vi "PNA3672B-H.vi"() -> ()   [LabVIEW 2018]
uses:
  <vilib>/Utility/file.llb/Write Delimited Spreadsheet (DBL).vi
panel:
  in  "Set Meter X":u16(ring) items=["PMMS field  0", "PPMS temp  1", "PPMS angle 2"]
  in  "Rate":dbl=50.0
  in  "Scan type":u16(ring)=1 items=["sweep  0", "liner  1"]
  in  "Int Rate (Oe/s)\nRate()":dbl=200.0 format="%#_13g"
  in  "Int Delay":dbl=5.0
  in  "Measurement Type":i32(ring)=2 items=["S11", "S12", "S21", "S22", "A", "B", "R1", "R2", "A/B", "B/A"]
  in  "Sweep Points (801)":i32=401
  in  "Stop Freq (26.4 E+9)":dbl=10000000000.0 format="%.2p"
  in  "Start Freq (10.0 E+6)":dbl=5000000000.0 format="%.2p"
  in  "?":enum32{"S-parameter", "Phase"}(tab)
  out "?":dbl[](graph)=[-5.13992176013, -5.77985062144, -7.16807133092, -9.42108029997, -10.1399493654, -8.71596720045, -7.83267897782, -7.42919537856, -6.76032356605, -6.18585704171, -5.97046539483, -5.73016109242, -5.37263627886, -5.1017928619, -5.00368082967, -5.17829909409, -5.80323496787, -7.15574927433, -8.9987014472, -9.38466845211, -8.49380537991, -7.97106763789, -7.32574501548, -6.50085765669, -6.07911357188, -5.85829530019, -5.55446508735, -5.36941855458, -5.36021729011, -5.31851913016, -5.5643037132, -6.25259294468, -7.43240745282, -9.04614952431, -9.99905930623, -9.4413228677, -8.04418422737, -6.84363600252, -6.40371174912, -6.24462050869, -5.56869109258, -4.87352825858, -4.66321212934, -4.69307312429, -4.7591466358, -5.14591077224, -5.89876799636, -7.07657010714, -8.54625263275, -9.49167159085, -9.24509469713, -8.19081925887, -7.18917811597, -6.67042363043, -6.07630869368, -5.34692013326, -4.941337791, -4.84078157888, -4.73147936533, -4.79218794585, -5.14409746704, -5.78112817858, -6.86212442292, -8.05457821576, -8.81261762726, -8.79759046484, -7.92763479317, -6.85071777851, -6.21538876741, -5.77195549778, -5.33268495617, -5.03854648325, -4.88320527288, -4.92756756489, -5.11628322032, -5.50972588621, -6.30511280642, -7.56416681135, -8.3419108514, -8.66657669285, -8.81033918175, -8.33720970709, -7.27317631141, -6.37575047564, -5.75176099873, -5.26236758865, -4.89247637429, -4.65199723878, -4.64290261895, -4.80678031934, -5.27987797209, -6.19570891325, -7.17215718437, -7.74510640519, -8.53976798715, -8.98978028998, -8.64998426925, -7.70133626893, -6.94492286579, -6.39681487173, -5.94202187224, -5.51750467546, -5.20454435892, -5.09708374418, -5.13935702712, -5.44519548006, -6.11037282184, -6.71822270524, -7.21836141914, -7.75556602746, -7.94679767326, -7.58810236429, -7.11458256386, -6.64461014107, -6.17815328806, -5.82869822125, -5.58855306212, -5.47932972608, -5.57017360045, -5.73509999009, -6.10279430727, -6.65628309091, -7.20691574144, -7.75099153049, -8.14236217319, -7.98342278217, -7.63567730066, -7.37171742701, -6.93968192443, -6.37024086203, -5.917649598, -5.55597456297, -5.30308721864, -5.25401060366, -5.39488001063, -5.74026002176, -6.23480440616, -6.7661133476, -7.41657074229, -7.91867432885, -8.02300874345, -8.08809276389, -7.99786036781, -7.59075128208, -7.08210024901, -6.64548196863, -6.30005305904, -6.11058253071, -6.07953628099, -6.16464230657, -6.4216011742, -6.75039933455, -7.09214315299, -7.52704057997, -7.86129689791, -7.85671742728, -7.68286255005, -7.41290778429, -7.08377575548, -6.76583315521, -6.51875926079, -6.34242015251, -6.29759006079, -6.28815023049, -6.49115089113, -6.90636491421, -7.42097777053, -7.82869609191, -8.25316429775, -8.57203674825, -8.66045753728, -8.58510840229, -8.34411171176, -8.02714571689, -7.70639713953, -7.43771426738, -7.29138512983, -7.25008195523, -7.33202806195, -7.54992861785, -7.91918366742, -8.29162811805, -8.70581027915, -9.12417570214, -9.40804943396, -9.52932859893, -9.52034892046, -9.35525338025, -9.1032378942, -8.86236246566, -8.66294128383, -8.56510147029, -8.56774273254, -8.68410230266, -8.89739073051, -9.14323997619, -9.40506155611, -9.67348671236, -9.91088070103, -10.0542110985, -10.1095993532, -10.0803215484, -9.93148871528, -9.72256956142, -9.5147582593, -9.31823788768, -9.17445611494, -9.08113535802, -9.05167488482, -9.03923798355, -9.03083138808, -8.97910059153, -8.88873008249, -8.75205020612, -8.56332184176, -8.38303089171, -8.22071675953, -8.1326945275, -8.05324942924, -8.05991169849, -8.05283861322, -8.16061412627, -8.29991125623, -8.47313413203, -8.57827792821, -8.65705773799, -8.67162556802, -8.6057904591, -8.47009108033, -8.25729780045, -8.0152070315, -7.7655926039, -7.57485266834, -7.4910467002, -7.5129644452, -7.59557810152, -7.73661469714, -7.87778576133, -7.99771913554, -8.13288701393, -8.32119654517, -8.46279170426, -8.35203711312, -8.15020651839, -7.88837024277, -7.57982328212, -7.34318110093, -7.19136752754, -7.15618430333, -7.21185640414, -7.36077780873, -7.56529300929, -7.83073868392, -8.06774468869, -8.2351880619, -8.33762695258, -8.31073052943, -8.14118362882, -7.90375456362, -7.61723861488, -7.2588078898, -6.98083255383, -6.72776846318, -6.63447620124, -6.71988359154, -6.77368052089, -7.11144857387, -7.37229013114, -7.68932033478, -7.98689247769, -8.19760417787, -8.28714274409, -8.23062581971, -8.04937534418, -7.79579768498, -7.49888178556, -7.14573710276, -6.8922594941, -6.68162816217, -6.62820636947, -6.6955037322, -6.78307910466, -7.05744034392, -7.40195880161, -7.7574756049, -8.08037713376, -8.15070297057, -8.18821061526, -8.11423800124, -8.14165480442, -7.82050654127, -7.70209407804, -7.46090411593, -7.38273407697, -7.28868801655, -7.2807538442, -7.37534790317, -7.51701471023, -7.62436761408, -7.74089685338, -7.80383275981, -7.78343031545, -7.69515063327, -7.53178482724, -7.31402064896, -7.10952415038, -6.93928420782, -6.83727474814, -6.81097857553, -6.86779731028, -6.98749866679, -7.1971793431, -7.38247926971, -7.54210372946, -7.63862857053, -7.6778904201, -7.62271286134, -7.51451127096, -7.34315098363, -7.14136947685, -6.96438816881, -6.79121451838, -6.69070621876, -6.65869471212, -6.6568027501, -6.72643653407, -6.75786124102, -6.84265238932, -6.87777149766, -6.88558318069, -6.83848750817, -6.77553827667, -6.73350349871, -6.65482701872, -6.61622596932, -6.6129050715, -6.66890540435, -6.75901895758, -6.87042004371, -6.99510404698, -7.12635533618, -7.23896129909, -7.3018797066, -7.30472334689, -7.2278149539, -7.12604877595, -6.99605011464, -6.87128470585, -6.7482182436, -6.68177936196, -6.64596095095, -6.67518331249, -6.72354301906, -6.76504258436, -6.82319955092, -6.88612600955, -6.96369683881, -6.96338059421, -6.94981925867, -6.96403414884, -7.03463520635, -7.05139105632, -7.06288523133, -7.13843539676, -7.23109085353, -7.37977824355, -7.53461754848, -7.69673249323, -7.72378467103, -7.5683548814, -7.38247183674, -7.21553067591, -7.04830148594, -6.7342671306, -6.48401257302, -6.32864044001, -6.26546650427, -6.27421138562, -6.39994502813, -6.65464294869, -7.02210039821, -7.43592259732, -7.79248421008, -7.98611288379, -7.936089008, -7.72371617285, -7.43734298033, -7.08800620268, -6.70804913045, -6.40077439135, -6.20272644312, -6.08472382437, -6.05534323724, -6.16756242594, -6.45803936543, -6.94832314698, -7.53318826156, -8.1920689104, -8.83012599835, -8.93751078087, -8.51422059906]
  in  "Format 1":string(combo)="IMAGinary"
  out "Sweep Time":dbl=0.19447074 format="%.2p"
  out "强度图":dbl[][](graph)
  out "?":dbl[](graph)=[32.7315489441, -56.8824930209, -156.803721114, 88.5947580109, -30.9871374098, -141.449771615, 121.640209048, 37.6741293404, -40.8852651853, -119.359692213, 163.750895669, 88.8384574151, 13.3240499463, -63.9260096883, -143.405981865, 133.50983641, 44.7073194162, -53.5440511171, -162.601840619, 79.6102257103, -33.2172204397, -129.587126545, 146.770832642, 66.0878076236, -13.5370500567, -90.5924606956, -167.123471558, 115.554059762, 38.2283746273, -41.0001051979, -124.5184635, 147.282505129, 51.2497788989, -55.3731568606, -169.072027126, 83.656838734, -12.3021295083, -102.452717622, 172.324212586, 94.0523173761, 18.2165179889, -60.6156999542, -140.290937488, 140.810952688, 60.5738116612, -22.7172481731, -109.652017526, 157.110661295, 55.5866667056, -53.048087914, -159.690576715, 102.426242104, 10.9688911141, -74.6158856148, -155.081353888, 124.521714604, 43.6872727344, -35.7101270301, -114.590575382, 164.575544825, 82.0901426192, -3.95730226738, -95.0285928659, 167.794680235, 63.4588246527, -41.3214166135, -139.542029674, 127.111889367, 38.4815112044, -45.3547081312, -126.698352397, 152.651043355, 72.8446050682, -7.32560497409, -87.954289903, -171.230817426, 102.154808567, 13.2571754957, -79.6451209514, 178.303953923, 74.3792037792, -23.0304688081, -115.678534016, 154.832081054, 69.078005824, -13.7902174538, -95.1617582494, -176.131266186, 102.595765505, 20.070955094, -64.77731603, -151.901641013, 120.060177573, 25.9178457946, -74.1552255377, -172.122975555, 94.1815920909, 2.03725084929, -87.9142000741, -174.423581853, 101.589486571, 18.9341666675, -63.971438346, -147.051928699, 128.678423861, 42.0808306788, -46.0050808644, -135.731355716, 130.13457169, 33.6068897418, -61.4897176925, -155.108417403, 113.175505949, 24.5315133942, -62.1326199724, -147.488272424, 128.115000927, 43.7882921958, -40.6090269269, -125.642775982, 147.354518001, 58.9206602667, -31.5941239859, -124.861969493, 141.766872237, 48.291882116, -45.4663429063, -136.890884056, 135.083717726, 47.7746115954, -38.6603639921, -124.258719066, 150.511571612, 65.2257451029, -20.5321047268, -107.529724429, 163.858540461, 72.6260181241, -20.7889524121, -113.818227096, 152.538492755, 58.8294740517, -31.932569054, -119.679705811, 153.414625818, 67.9360203075, -16.761149864, -101.241236752, 174.044379129, 88.3204159639, 0.878356230139, -88.3268956559, 179.63752201, 85.3637790641, -9.034868342, -103.096223064, 163.658409742, 72.8031961431, -15.6688017348, -102.22000084, 172.884816589, 88.5456131454, 4.55185396442, -80.2707904752, -166.719177803, 105.182195151, 16.096076312, -75.3026072059, -168.714844573, 97.6383537905, 4.33654879439, -87.7067545736, -177.84505287, 93.8380017628, 6.97761796918, -78.9002782548, -164.400040415, 110.116141956, 24.0091146464, -62.9948301844, -150.732269265, 120.632831154, 30.5535960961, -60.2411898127, -151.292645694, 117.497721205, 26.9689156873, -62.5301818212, -151.367772947, 120.685035314, 33.3394512614, -53.5091290058, -140.068434299, 133.595476642, 47.2881570478, -39.0864346002, -125.960768837, 146.612134326, 58.7129453948, -29.8143369144, -118.986171156, 151.549019718, 61.9477483812, -27.6598757887, -116.976616287, 154.302945475, 66.1878564391, -21.2904270435, -108.127149698, 165.52171244, 79.4590872768, -6.83103821612, -93.6121690666, 178.732349126, 90.3652078735, 1.14449863919, -88.5963134199, -178.65967342, 91.3537131772, 1.69568242194, -87.743176037, -176.928296806, 94.3550205229, 6.14869585327, -81.7831524664, -169.539688075, 102.802172688, 15.0397411523, -72.8651220086, -160.916924229, 110.823595481, 22.527364207, -65.9275903187, -154.288949487, 117.446350182, 28.9943452624, -59.7324147838, -148.897831038, 121.577481918, 31.6490376728, -58.2592650543, -147.677831112, 123.372313971, 35.0181759661, -52.4179118064, -139.26608448, 134.01427806, 47.4191105099, -39.5141347671, -126.836073187, 144.949439688, 55.7351697066, -34.3928698653, -125.099446067, 143.632754958, 52.5752734821, -37.7294449644, -127.148944827, 144.53035721, 57.5778533047, -28.887570595, -114.999609647, 158.525366628, 71.0429767896, -15.3772796346, -103.919515773, 166.689371892, 77.0093180077, -13.7911821267, -104.825362398, 164.200014669, 74.3696417703, -14.7668942558, -102.967824914, 169.411234659, 82.6122419887, -4.39400690011, -91.4543478077, -178.76858485, 93.3771862952, 4.85591617141, -84.3294425775, -173.865576593, 96.3465827134, 6.2490852757, -83.2265580877, -173.015984117, 97.78007546, 8.28655359163, -79.76381321, -167.927920395, 105.464735796, 17.261076543, -70.0043839303, -157.791686994, 114.069074987, 25.2581831541, -63.7608616106, -153.623185239, 116.145683725, 25.8986335399, -64.2331220915, -154.057904631, 116.747887891, 28.1083515487, -59.9530342147, -147.477795048, 125.430845568, 38.358901893, -48.7756883964, -136.513013638, 135.090000778, 45.9410900506, -44.132522883, -134.81386025, 134.272943326, 43.463402508, -47.1014527938, -136.910600874, 134.009988341, 45.6836835135, -41.9002560197, -129.524645098, 143.209830004, 55.3766093333, -32.4089929655, -121.157084902, 149.743492126, 60.2247754669, -29.3814603663, -118.881768282, 151.742455687, 62.7529965091, -25.7990392292, -114.353341921, 157.350941943, 68.9119611723, -19.6248853555, -108.53843891, 162.242639238, 72.8768930287, -16.4662361825, -105.666386314, 165.419060839, 76.7648920544, -11.5379476172, -99.5758100655, 172.435108019, 84.1025390815, -4.88019096974, -94.3024874425, 175.738534312, 85.5960595678, -4.7695105397, -94.9315233658, 175.485146261, 86.9188499232, -0.563780453117, -87.6986696312, -174.426390626, 99.1825213591, 13.1552601395, -74.0907708672, -162.246232711, 108.15987703, 17.2417782382, -74.8265647472, -167.397054628, 100.744515615, 9.42910460872, -80.8444801244, -169.303652166, 104.659034338, 19.8043132765, -65.0554301395, -149.709685307, 125.555931464, 40.1202806793, -46.5671247267, -134.968163745, 134.5694261, 41.8189582943, -52.9338270423, -148.539509551, 116.764065214, 24.1899149115, -65.4304007989, -152.041950572, 122.95863872, 39.038287934, -44.0062424284, -126.556835392, 150.597800658, 66.9189093569, -18.4084130856, -105.815690398, 163.407074758, 67.8515876273, -29.9904541232, -128.522871427, 135.807686]
  in  "Format 2":string(combo)="PHASe"
  out "强度图 2":dbl[][](graph)
  out "VISA 2":refnum<visa-resource-name>="GPIB0::16::INSTR"
  out "Time(s)":dbl=21.755
  out "Current H (Oe)":dbl=19.0 format="%.4g"
  in  "File":string="Hello"
  in  "Directory":string="D:\\ff"
  out "file":path=path "E:/ff/Hello@_100ms_1.txt"
  in  "wait":u32=400
  out "Hset":dbl[](array[numeric])=[14.0, 14.5, 15.0, 15.5, 16.0, 16.5, 17.0, 17.5, 18.0, 18.5, 19.0]
  in  "L/S":enum32{"Loop", "Scan"}(radio)=enum."Scan"
  in  "停止":bool
  in  "Hpara":dbl[][](array[numeric])=[[-1000.0, 1000.0, 10.0], [0.0, 0.0, 0.0], [0.0, 0.0, 0.0], [0.0, 0.0, 0.0], [0.0, 0.0, 0.0], [0.0, 0.0, 0.0], [0.0, 0.0, 0.0], [0.0, 0.0, 0.0], [0.0, 0.0, 0.0], [0.0, 0.0, 0.0], [0.0, 0.0, 0.0], [0.0, 0.0, 0.0], [0.0, 0.0, 0.0]] caption="Hi(Oe)     Hf(Oe)   Steps"
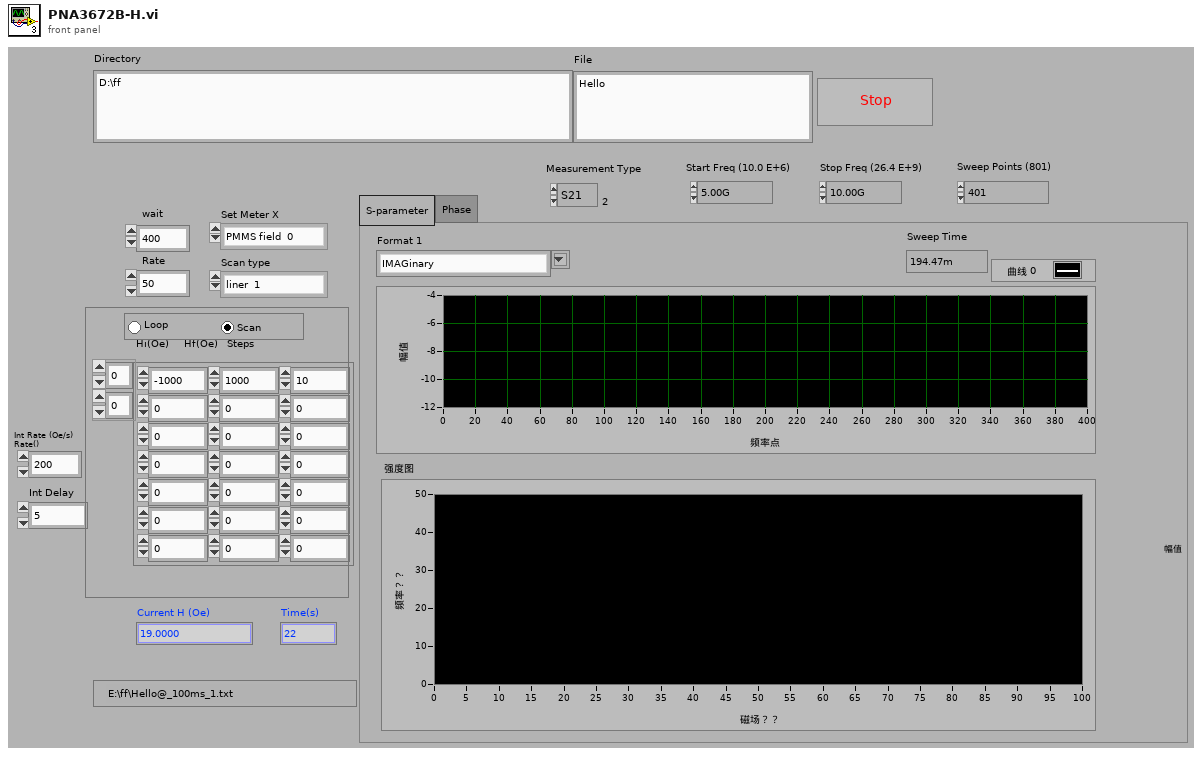
[diagram p1: front panel]
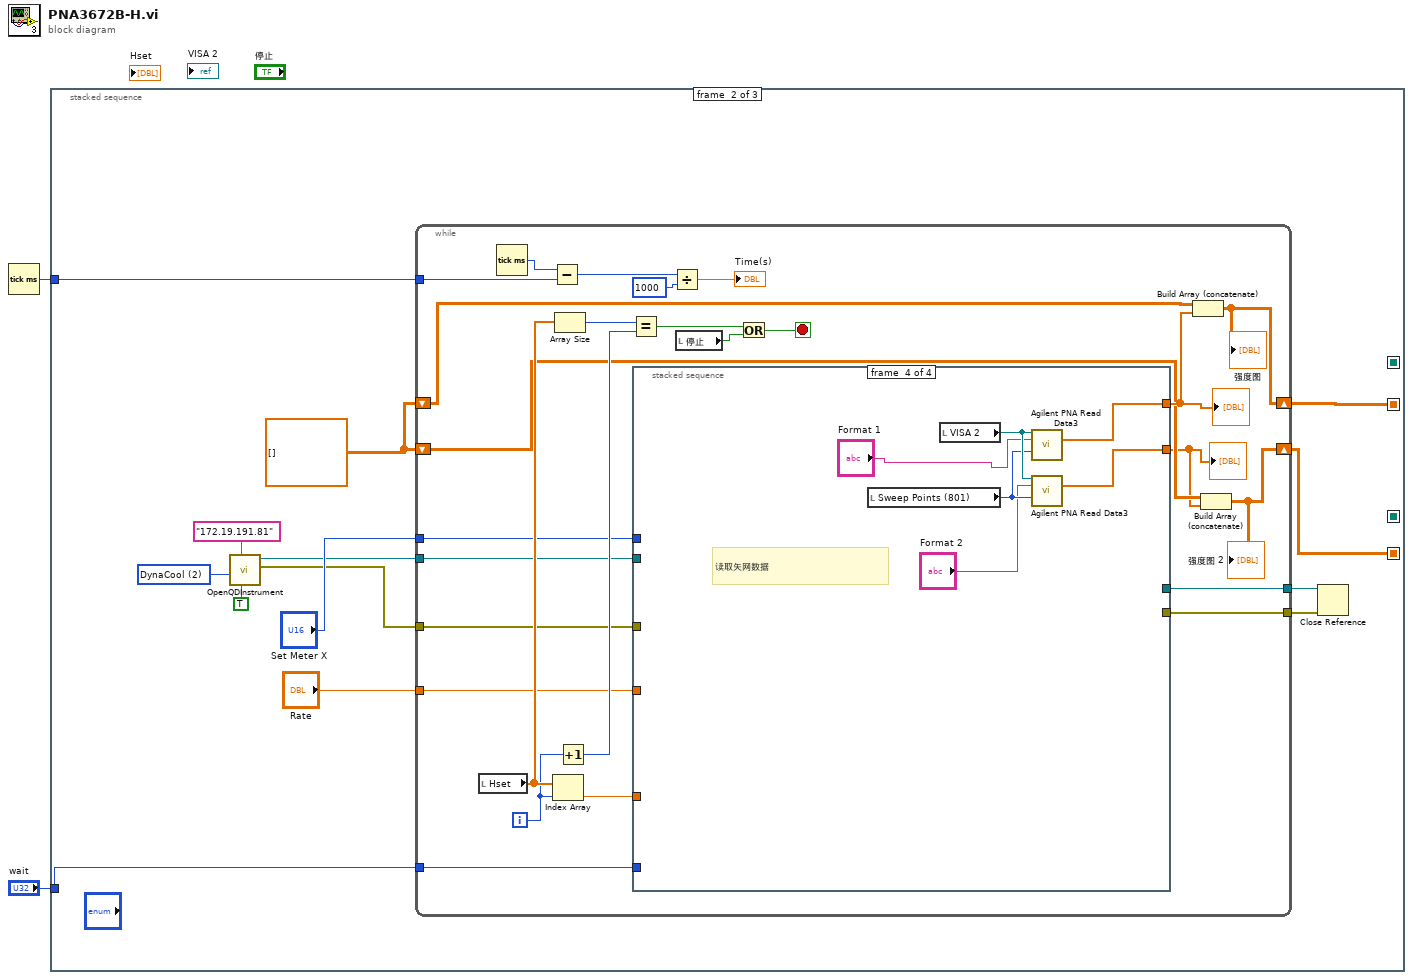
[diagram p0: block diagram]
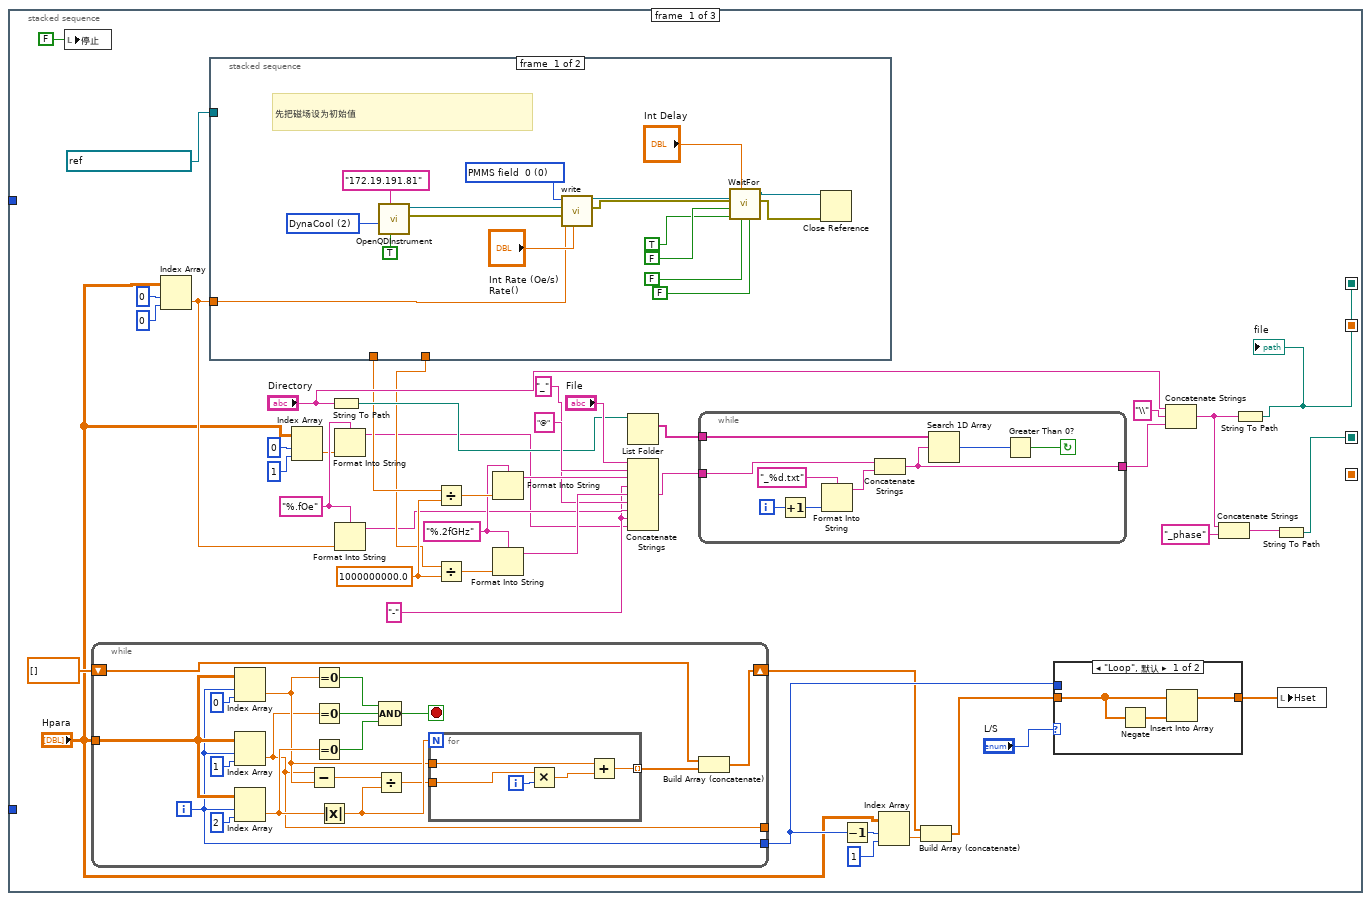
[diagram p2: hidden frame]
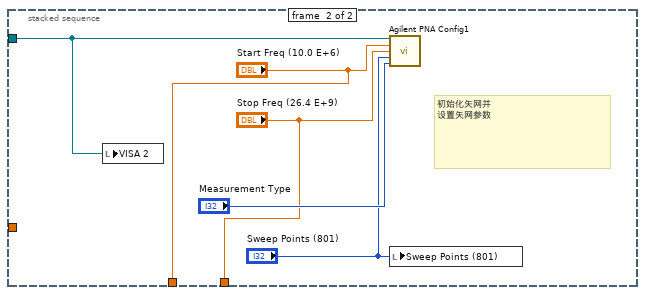
[diagram p3: hidden frame]
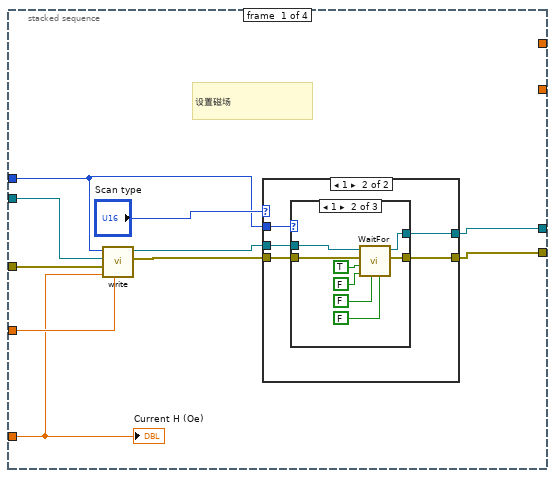
[diagram p5: hidden frame]
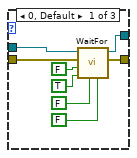
[diagram p7: hidden frame]
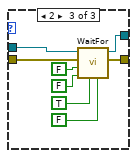
[diagram p8: hidden frame]
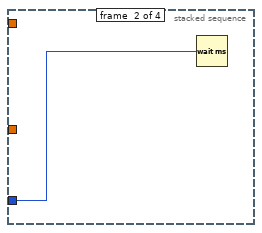
[diagram p9: hidden frame]
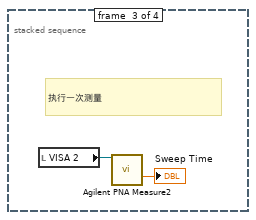
[diagram p10: hidden frame]
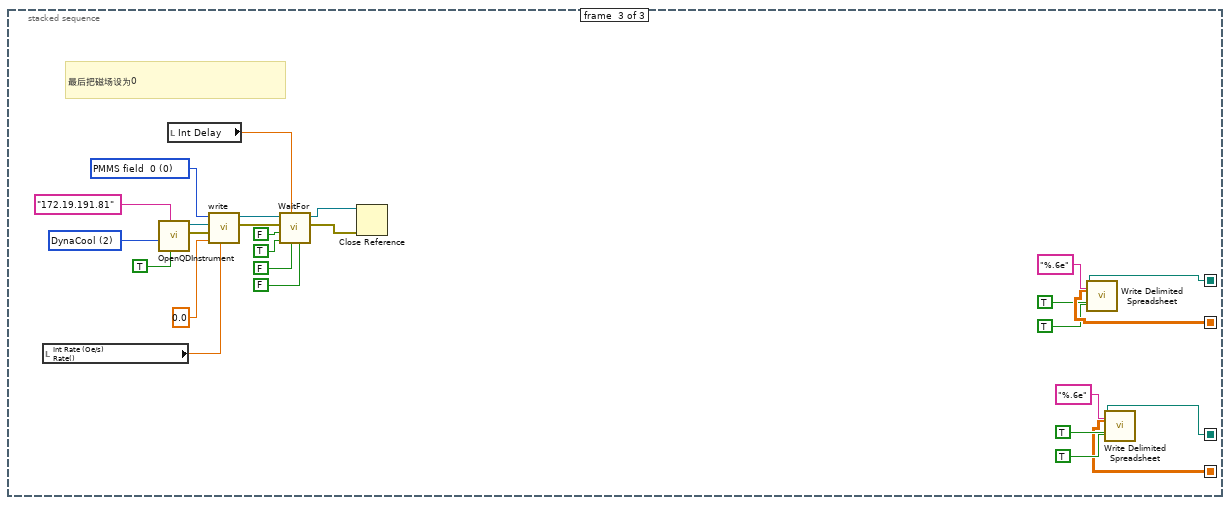
[diagram p11: hidden frame]
diagram:
  n1 = Tick Count (ms)() -> (millisecond timer value=w2:u32)
  n2 = stacked-sequence {
    seq-local: [_ w115 _] -> [_ _ w219]
    seq-local: [w35 _ _] -> [_ _ w221]
    seq-local: [w3 _ _] -> [_ _ w196]
    seq-local: [_ w105 _] -> [_ _ w195]
    tunnel: w2 -> [_ w118 _]
    tunnel: "wait" -> [_ w117 _]
    frame #0 {
      w9 = "%.fOe" ("格式字符串")
      w13 = "-" ("字符串")
      w20 = 1000000000.0 ("y")
      w21 = "%.2fGHz" ("格式字符串")
      n3 = local write "停止"(FALSE ("停止")) -> ()
      n4 = while {
        tunnel: "Hpara" -> [w92]
        shift-right: [w85] -> w29
        shift-left: dbl[] [] -> [w84]
        tunnel: [w83] -> _
        tunnel: [w82] -> w31
        i -> [w82]
        stop <- w96 stop-if-true
        n5 = Index Array(array=w92, index (row)=w82, index (col)=0 ("禁用的索引 (col)")) -> (element=w87:dbl)
        n6 = Index Array(array=w92, index (row)=w82, index (col)=1 ("禁用的索引 (col)")) -> (element=w83:dbl)
        n7 = Index Array(array=w92, index (row)=w82, index (col)=2 ("禁用的索引 (col)")) -> (element=w91:dbl)
        n8 = Subtract(x=w83, y=w87) -> (x-y=w90:dbl)
        n9 = Equal To 0?(x=w87) -> (x = 0?=w99:bool)
        n10 = Equal To 0?(x=w83) -> (x = 0?=w98:bool)
        n11 = Equal To 0?(x=w91) -> (x = 0?=w97:bool)
        n12 = Absolute Value(x=w91) -> (abs(x)=w89:dbl)
        n13 = Divide(x=w90, y=w89) -> (x/y=w88:dbl)
        n14 = Compound Arithmetic op=AND(w99, w98, w97) -> (w96:bool)
        n15 = for {
          N: w89 -> [_]
          tunnel: [w104] -> w86 mode=indexing
          tunnel: w88 -> [w101]
          tunnel: w87 -> [w100]
          i -> [w103]
          n16 = Multiply(x=w101, y=w103) -> (x*y=w102:dbl)
          n17 = Add(x=w100, y=w102) -> (x+y=w104:dbl)
        }
        n18 = Build Array (concatenate)(w84, w86) -> (w85:dbl[])
      }
      n19 = Index Array(array="Hpara", index (row)=0 ("索引 (行)"), index (col)=0 ("禁用的索引 (col)")) -> (element=w15:dbl)
      n20 = stacked-sequence {
        tunnel: refnum<visa-resource-name> "GPIB0::16::INSTR" ("VISA资源名称") -> [_ w66]
        tunnel: w15 -> [w49 _]
        tunnel: [_ "Start Freq (10.0 E+6)"] -> w24
        tunnel: [_ "Stop Freq (26.4 E+9)"] -> w19
        frame #0 {
          w58 = u16 0 items=["PMMS field  0", "PPMS temp  1", "PPMS angle 2"] ("Set Meter")
          w61 = 2 items=["PPMS", "VersaLab", "DynaCool", "SVSM"] ("Instrument\nType")
          # "先把磁场设为初始值"
          n21 = call "OpenQDInstrument.vi"("Remote"=TRUE, "IP Address"="172.19.191.81", "Instrument Type"=w61) -> ("error out"=w59:errorcluster, "Instrument Ref"=w60:refnum<k24>)  [unwired: 5 in]
          n22 = call "write.vi"("Rate"="Int Rate (Oe/s)\nRate()", "value"=w49, "error in (no error)"=w59, "Instrument Ref In"=w60, "Set Meter"=w58) -> ("error out"=w56:errorcluster, "Instrument Ref Out"=w55:refnum<k24>)  [unwired: 5 in]
          n23 = call "WaitFor.vi"("Wait For Chamber"=FALSE, "Wait For Position"=FALSE, "Delay"="Int Delay", "Wait For Field"=TRUE, "Wait For Temperature"=FALSE, "error in (no error)"=w56, "Instrument Ref In"=w55) -> ("error out"=w47:errorcluster, "Instrument Ref Out"=w48:refnum<k24>)  [unwired: 3 in]
          n24 = Close Reference(reference=w48, error in (no error)=w47) -> ()  [unwired: 1 out]
        }
        frame #1 {
          # "初始化矢网并\n设置矢网参数"
          n25 = local write "VISA 2"(w66) -> ()
          n26 = call "Agilent PNA Config1.vi"("VISA session"=w66, "Start Freq (10.0 E+6)"="Start Freq (10.0 E+6)", "Stop Freq (26.4 E+9)"="Stop Freq (26.4 E+9)", "Sweep Points (801)"="Sweep Points (801)", "Measurement Type (0: S11)"="Measurement Type") -> ()  [unwired: 9 in, 2 out]
          n27 = local write "Sweep Points (801)"("Sweep Points (801)") -> ()
        }
      }
      n28 = Index Array(array="Hpara", index (row)=0 ("索引 (行)"), index (col)=1 ("禁用的索引 (col)")) -> (element=w8:dbl)
      n29 = String To Path(string="Directory") -> (path=w41:path)
      n30 = Format Into String(format string=w9, w8) -> (resulting string=w7:string)  [unwired: 2 in, 1 out]
      n31 = Format Into String(format string=w9, w15) -> (resulting string=w14:string)  [unwired: 2 in, 1 out]
      n32 = Divide(x=w24, y=w20) -> (x/y=w23:dbl)
      n33 = Divide(x=w19, y=w20) -> (x/y=w18:dbl)
      n34 = Format Into String(format string=w21, w23) -> (resulting string=w22:string)  [unwired: 2 in, 1 out]
      n35 = Format Into String(format string=w21, w18) -> (resulting string=w17:string)  [unwired: 2 in, 1 out]
      n36 = List Folder(path=w41) -> (filenames=w40:string[])  [unwired: 3 in, 3 out]
      n37 = Concatenate Strings("File", "@" ("string"), w22, w13, w17, "_" ("字符串"), w14, w13, w7) -> (w39:string)
      n38 = while {
        tunnel: w40 -> [w77]
        tunnel: w39 -> [w69]
        tunnel: [w70] -> w36
        i -> [w72]
        stop <- w75 continue-if-true
        n39 = Increment(x=w72) -> (x+1=w71:i32)
        n40 = Format Into String(format string="_%d.txt", w71) -> (resulting string=w73:string)  [unwired: 2 in, 1 out]
        n41 = Concatenate Strings(w69, w73) -> (w70:string)
        n42 = Search 1D Array(1D array=w77, element=w70) -> (index of element=w76:i32)  [unwired: 1 in]
        n43 = Greater Than 0?(x=w76) -> (x > 0?=w75:bool)
      }
      n44 = Decrement(x=w31) -> (x-1=w26:i32)
      n45 = Index Array(array="Hpara", index (row)=w26, index (col)=1 ("禁用的索引 (col)")) -> (element=w30:dbl)
      n46 = Build Array (concatenate)(w29, w30) -> (w28:dbl[])
      n47 = case shown="\"Loop\", 默认" "L/S" {
        tunnel: w28 -> [w79 w81]
        tunnel: [w80 w81] -> w27
        tunnel: w31 -> [_ _]
        frame "Loop", Default {
          n48 = Negate(x=w79) -> (-x=w78:dbl[])
          n49 = Insert Into Array(array=w79, new element=w78) -> (w80:dbl[])  [unwired: 1 in]
        }
        frame "Scan" {
        }
      }
      n50 = Concatenate Strings("Directory", "\\" ("string"), w36) -> (w6:string)
      n51 = Concatenate Strings(w6, "_phase" ("字符串")) -> (w5:string)
      n52 = String To Path(string=w6) -> (path=w35:path)
      "file" <- w35
      n53 = String To Path(string=w5) -> (path=w3:path)
      n54 = local write "Hset"(w27) -> ()
    }
    frame #1 {
      w112 = 2 items=["PPMS", "VersaLab", "DynaCool", "SVSM"] ("Instrument\nType")
      w116 = dbl[][] []
      n55 = call "OpenQDInstrument.vi"("Remote"=TRUE, "IP Address"="172.19.191.81", "Instrument Type"=w112) -> ("error out"=w109:errorcluster, "Instrument Ref"=w108:refnum<k24>)  [unwired: 5 in]
      n56 = while "前一次磁场" {
        shift-right: [w120] -> w115
        shift-left: w116 -> [w130]
        shift-right: [w119] -> w105
        shift-left: w116 -> [w128]
        tunnel: w118 -> [w137]
        tunnel: w117 -> [w132]
        tunnel: "Rate" -> [w126]
        tunnel: "Set Meter X" -> [w125]
        tunnel: w109 -> [w124]
        tunnel: w108 -> [w123]
        tunnel: [w122] -> w107
        tunnel: [w121] -> w106
        i -> [w138]
        stop <- w144 stop-if-true
        n57 = local read "Hset"() -> (w139:dbl[])
        n58 = Tick Count (ms)() -> (millisecond timer value=w136:u32)
        n59 = Subtract(x=w136, y=w137) -> (x-y=w135:u32)
        n60 = Index Array(array=w139, index=w138) -> (element=w131:dbl)
        n61 = Array Size(array=w139) -> (size(s)=w142:i32)
        n62 = Increment(x=w138) -> (x+1=w141:i32)
        n63 = Equal?(x=w142, y=w141) -> (x = y?=w140:bool)
        n64 = stacked-sequence {
          tunnel: [_ _ _ w192] -> w129
          tunnel: w131 -> [w150 _ _ _]
          tunnel: w132 -> [_ w186 _ _]
          tunnel: [_ _ _ w191] -> w127
          tunnel: w126 -> [w151 _ _ _]
          tunnel: w125 -> [w149 _ _ _]
          tunnel: w124 -> [w148 _ _ _]
          tunnel: w123 -> [w147 _ _ _]
          tunnel: [w146 _ _ _] -> w122
          tunnel: [w145 _ _ _] -> w121
          frame #0 {
            # "设置磁场"
            n65 = call "write.vi"("Rate"=w151, "value"=w150, "error in (no error)"=w148, "Instrument Ref In"=w147, "Set Meter"=w149) -> ("error out"=w153:errorcluster, "Instrument Ref Out"=w154:refnum<k24>)  [unwired: 5 in]
            n66 = case shown="1" "Scan type" {
              tunnel: w154 -> [w156 w161]
              tunnel: w153 -> [w155 w160]
              tunnel: w149 -> [_ w159]
              tunnel: [w156 w158] -> w146
              tunnel: [w155 w157] -> w145
              frame 0, Default {
              }
              frame 1 {
                n67 = case shown="1" w159 {
                  tunnel: w161 -> [w169 w177 w185]
                  tunnel: w160 -> [w168 w176 w184]
                  tunnel: [w163 w171 w179] -> w158
                  tunnel: [w162 w170 w178] -> w157
                  frame 0, Default {
                    n68 = call "WaitFor.vi"("Wait For Chamber"=FALSE, "Wait For Position"=FALSE, "Wait For Field"=TRUE, "Wait For Temperature"=FALSE, "error in (no error)"=w168, "Instrument Ref In"=w169) -> ("error out"=w162:errorcluster, "Instrument Ref Out"=w163:refnum<k24>)  [unwired: 4 in]
                  }
                  frame 1 {
                    n69 = call "WaitFor.vi"("Wait For Chamber"=FALSE, "Wait For Position"=FALSE, "Wait For Field"=FALSE, "Wait For Temperature"=TRUE, "error in (no error)"=w176, "Instrument Ref In"=w177) -> ("error out"=w170:errorcluster, "Instrument Ref Out"=w171:refnum<k24>)  [unwired: 4 in]
                  }
                  frame 2 {
                    n70 = call "WaitFor.vi"("Wait For Chamber"=FALSE, "Wait For Position"=TRUE, "Wait For Field"=FALSE, "Wait For Temperature"=FALSE, "error in (no error)"=w184, "Instrument Ref In"=w185) -> ("error out"=w178:errorcluster, "Instrument Ref Out"=w179:refnum<k24>)  [unwired: 4 in]
                  }
                }
              }
            }
            "Current H (Oe)" <- w150
          }
          frame #1 {
            n71 = Wait (ms)(milliseconds to wait=w186) -> ()  [unwired: 1 out]
          }
          frame #2 {
            # "执行一次测量"
            n72 = local read "VISA 2"() -> (w188:refnum<visa-resource-name>)
            n73 = call "Agilent PNA Measure2.vi"("VISA session"=w188) -> ("Sweep Time"=→"Sweep Time":dbl)  [unwired: 12 in, 2 out]
          }
          frame #3 {
            # "读取矢网数据"
            n74 = local read "Sweep Points (801)"() -> (w193:i32)
            n75 = local read "VISA 2"() -> (w194:refnum<visa-resource-name>)
            n76 = call "Agilent PNA Read Data3.vi"("VISA session"=w194, "Format"="Format 1", "Sample Count (401)"=w193) -> ("Data"=w192:dbl[])  [unwired: 10 in, 2 out]
            n77 = call "Agilent PNA Read Data3.vi"("VISA session"=w194, "Format"="Format 2", "Sample Count (401)"=w193) -> ("Data"=w191:dbl[])  [unwired: 10 in, 2 out]
          }
        }
        "?" <- w127
        "?" <- w129
        n78 = Divide(x=w135, y=u32 1000) -> (x/y=→"Time(s)":dbl)
        n79 = local read "停止"() -> (w143:bool)
        n80 = Or(x=w140, y=w143) -> (x .or. y?=w144:bool)
        n81 = Build Array (concatenate)(w130, w129) -> (w120:dbl[][])
        "强度图" <- w120
        n82 = Build Array (concatenate)(w128, w127) -> (w119:dbl[][])
        "强度图 2" <- w119
      }
      n83 = Close Reference(reference=w107, error in (no error)=w106) -> ()  [unwired: 1 out]
    }
    frame #2 {
      w211 = u16 0 items=["PMMS field  0", "PPMS temp  1", "PPMS angle 2"] ("Set Meter")
      w214 = 2 items=["PPMS", "VersaLab", "DynaCool", "SVSM"] ("Instrument\nType")
      # "最后把磁场设为0"
      n84 = local read "Int Rate (Oe/s)\nRate()"() -> (w201:dbl)
      n85 = call "OpenQDInstrument.vi"("Remote"=TRUE, "IP Address"="172.19.191.81", "Instrument Type"=w214) -> ("error out"=w212:errorcluster, "Instrument Ref"=w213:refnum<k24>)  [unwired: 5 in]
      n86 = local read "Int Delay"() -> (w200:dbl)
      n87 = call "write.vi"("Rate"=w201, "value"=0.0, "error in (no error)"=w212, "Instrument Ref In"=w213, "Set Meter"=w211) -> ("error out"=w210:errorcluster, "Instrument Ref Out"=w209:refnum<k24>)  [unwired: 5 in]
      n88 = call "WaitFor.vi"("Wait For Chamber"=FALSE, "Wait For Position"=FALSE, "Delay"=w200, "Wait For Field"=TRUE, "Wait For Temperature"=FALSE, "error in (no error)"=w210, "Instrument Ref In"=w209) -> ("error out"=w203:errorcluster, "Instrument Ref Out"=w204:refnum<k24>)  [unwired: 3 in]
      n89 = Close Reference(reference=w204, error in (no error)=w203) -> ()  [unwired: 1 out]
      n90 = call-poly <vilib>:"Write Delimited Spreadsheet.vi"("file path (dialog if empty)"=w221, "format (%.3f)"="%.6e", "2D data"=w219, "append to file? (new file:F)"=TRUE, "transpose? (no:F)"=TRUE) -> ()  [unwired: 9 in, 2 out]
      n91 = call-poly <vilib>:"Write Delimited Spreadsheet.vi"("file path (dialog if empty)"=w196, "format (%.3f)"="%.6e", "2D data"=w195, "append to file? (new file:F)"=TRUE, "transpose? (no:F)"=TRUE) -> ()  [unwired: 9 in, 2 out]
    }
  }
